vi "AutoSetIntakeDemands.vi"(7 "IntakeDown":bool, 8 "error in (no error)":errorcluster, 9 "intakeUpperDemand":dbl, 10 "intakeLowerDemand":dbl, 11 "turntableDemand":dbl) -> ()   [LabVIEW 2020]
panel:
  out "error out":errorcluster
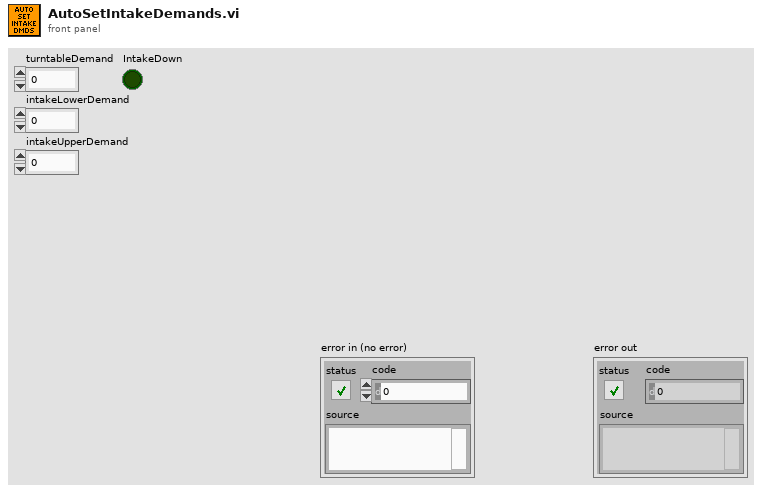
[diagram p1: front panel]
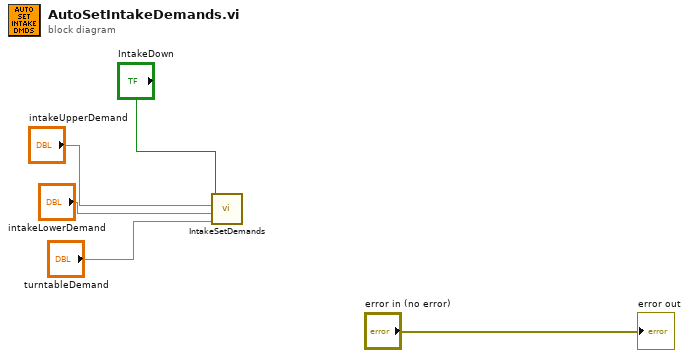
[diagram p0: block diagram]
diagram:
  n1 = call "IntakeSetDemands.vi"("turntableDemand"="turntableDemand", "intakeLowerDemand"="intakeLowerDemand", "intakeUpperDemand"="intakeUpperDemand", "IntakeDown"="IntakeDown") -> ()  [unwired: 8 in]
  "error out" <- "error in (no error)"
